vi "max_min_hold _2(SubVI).vi"(11 "theta":dbl) -> (2 "theta_min":dbl, 3 "theta_max":dbl)   [LabVIEW 2013]
uses:
  <vilib>/Simulation/Implementation/Shared/SIMSCR Execution Mode.ctl
  <vilib>/Simulation/Scripting/Companion Diagram/SimConfigNode/SimParams.ctl
  <vilib>/Simulation/Scripting/Companion Diagram/SimConfigNode/_simSolvers.ctl
  <vilib>/Simulation/Param Hierarchy/Typedefs/SIMPH Param Control Actions.ctl
  <vilib>/Simulation/Implementation/Shared/NILVSim_ParamChanged.vi
  <vilib>/Simulation/Implementation/Shared/NILVSIM_BeginStep.vi
  <vilib>/Simulation/ContinuousLinear/Implementation/NILVSim Zero Cross Detect.llb/SIM zero cross detect (scalar).vi
  <vilib>/Simulation/Utility/Implementation/NILVSim Memory.llb/NILVSim Memory (core).vi
  <vilib>/Simulation/Implementation/Shared/SIM Is Init or Final Stage.vi
  <vilib>/Simulation/Implementation/Shared/NILVSim_Manager.vi
  <vilib>/Simulation/Implementation/Shared/NILVSim_FinalizeModel.vi
  <vilib>/Simulation/Implementation/Shared/SIM Unbundle Sim Info.vi
  <vilib>/Utility/error.llb/Clear Errors.vi
  <vilib>/Simulation/Implementation/Shared/NILVSim_GetModelError.vi
  <vilib>/Simulation/Implementation/Shared/SIM SimErrorHandler.vi
  <vilib>/Simulation/Implementation/Shared/SIM Bundle Sim Info.vi
  <vilib>/Simulation/Implementation/Shared/SIMSH Read Queue.vi
  <vilib>/Simulation/Implementation/Shared/NILVSim_Initialize.vi
  <vilib>/Simulation/Utility/Implementation/NILVSim Get Time and IsAcceptedStep.vi
  <vilib>/Simulation/Scripting/Companion Diagram/SimConfigNode/SimDog.xnode
  <vilib>/Simulation/Implementation/XNodeFramework/SimXNode/SimX.xnode
  <vilib>/Simulation/Implementation/Shared/NI_SIM_Implementation.lvlib
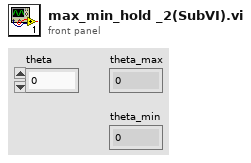
[diagram p1: front panel]
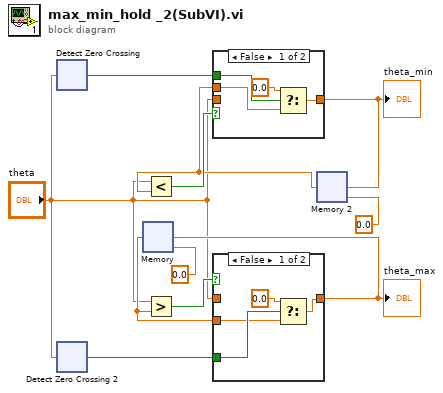
[diagram p0: block diagram]
diagram:
  n1 = xnode "Detect Zero Crossing"("input"="theta") -> ("crossed?"=w9:bool)  [unwired: 4 in]
  n2 = xnode "Detect Zero Crossing 2"("input"="theta") -> ("crossed?"=w1:bool)  [unwired: 4 in]
  n3 = xnode "Memory"("input"=w7, "initial value"=0.0) -> ("output"=w8:dbl)  [unwired: 4 in]
  n4 = Greater?(x="theta", y=w8) -> (0:w11:bool)
  n5 = case shown="False" w11 {
    tunnel: "theta" -> [_ w16]
    tunnel: [w15 w16] -> w7
    tunnel: w8 -> [w12 _]
    tunnel: w1 -> [w14 _]
    frame False {
      n6 = Select(t=0.0, s=w14, f=w12) -> (s? t:f=w15:dbl)
    }
    frame True {
    }
  }
  "theta_max" <- w7
  n7 = Less?(x="theta", y=w3) -> (x < y?=w10:bool)
  n8 = case "Case Structure 2" shown="False" w10 {
    tunnel: "theta" -> [_ w21]
    tunnel: [w20 w21] -> w5
    tunnel: w3 -> [w17 _]
    tunnel: w9 -> [w18 _]
    frame False {
      n9 = Select ("Select 2")(t=0.0 ("t 2"), s=w18, f=w17) -> (s? t:f=w20:dbl)
    }
    frame True {
    }
  }
  "theta_min" <- w5
  n10 = xnode "Memory 2"("input"=w5, "initial value"=0.0 ("initial value 2")) -> ("output"=w3:dbl)  [unwired: 4 in]
